vi "Write channel mapping.vi"(8 "error in (no error)":errorcluster, 11 "?":T1) -> (0 "error out":errorcluster)   [LabVIEW 2017]
uses:
  Controls/Testscreen_Input cluster.ctl
  <vilib>/addons/database/Connection.llb/Conn ObjectReference.ctl
  <vilib>/Utility/file.llb/Write Delimited Spreadsheet (string).vi
  <vilib>/addons/database/NI_Database_API.lvlib
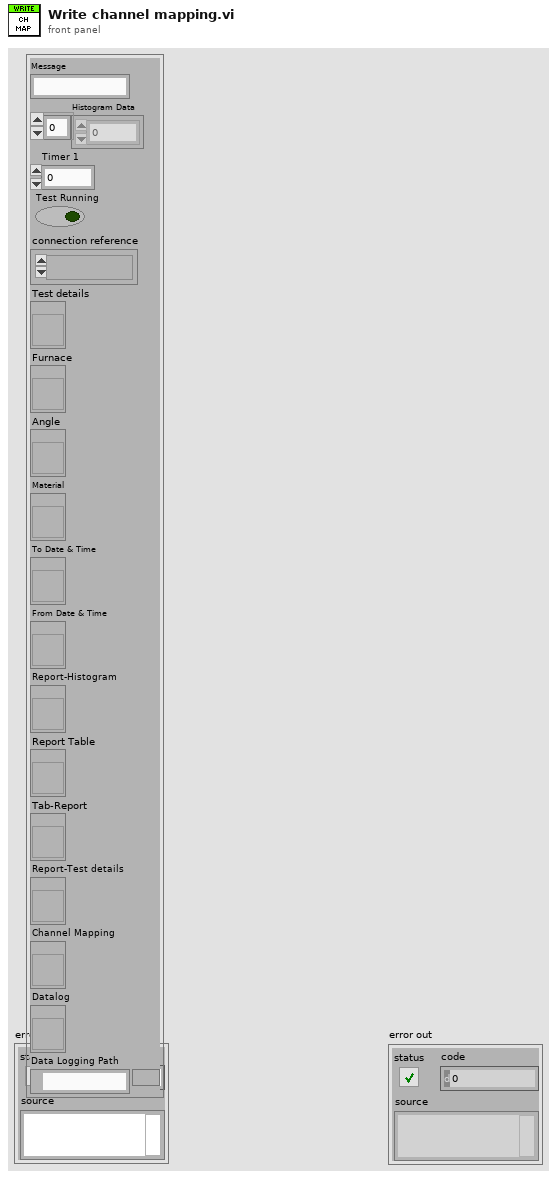
[diagram p1: front panel]
types:
  T1 = typedef "Testscreen_Input cluster.ctl" = cluster{"Message":string, "Histogram Data":i32[], "Timer 1":u32, "Test Running":bool, "connection reference":T2, "Test details":refnum<vi>, "Furnace":refnum<vi>, "Angle":refnum<vi>, "Material":refnum<vi>, "To Date & Time":refnum<vi>, "From Date & Time":refnum<vi>, "Report-Histogram":refnum<vi>, "Report Table":refnum<vi>, "Tab-Report":refnum<vi>, "Report-Test details":refnum<vi>, "Channel Mapping":refnum<vi>, "Datalog":refnum<vi>, "Data Logging Path":path}
  T2 = typedef "NI_Database_API.lvlib/Conn ObjectReference.ctl" = refnum<k1>
  T3 = cluster{"Channel Name":string, " Physical Channel":string, "Selecion?":bool}[]
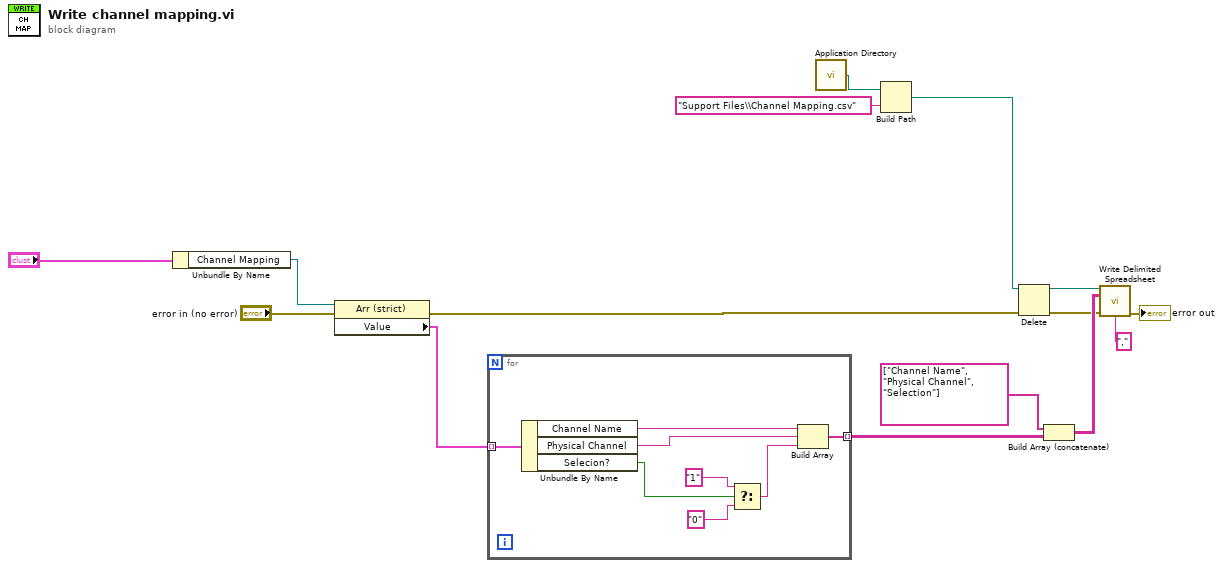
[diagram p0: block diagram]
diagram:
  n1 = Unbundle By Name("?") -> ("Channel Mapping"=w14:refnum<vi>)
  n2 = property class="Arr (strict)"(reference=w14, error in="error in (no error)") -> (error out=w2:errorcluster, "Value"=w12:T3)  [unwired: 1 out]
  n3 = for {
    tunnel: w12 -> [w23] mode=indexing
    tunnel: [w16] -> w10 mode=indexing
    n4 = Unbundle By Name(w23) -> ("Channel Name"=w19:string, "Physical Channel"=w18:string, "Selecion?"=w22:bool)
    n5 = Select(t="1", s=w22, f="0") -> (s? t:f=w17:string)
    n6 = Build Array(w19, w18, w17) -> (w16:string[])
  }
  n7 = call <vilib>:"Application Directory.vi"() -> ("Application Directory"=w9:path)
  n8 = Build Path(base path=w9, name or relative path="Support Files\\Channel Mapping.csv") -> (appended path=w4:path)
  n9 = Delete(path (use dialog)=w4, error in=w2) -> (deleted path=w3:path, error out=w1:errorcluster)  [unwired: 3 in, 1 out]
  n10 = Build Array (concatenate)(string[] ["Channel Name", "Physical Channel", "Selection"], w10) -> (w7:string[][])
  n11 = call-poly <vilib>:"Write Delimited Spreadsheet.vi"("file path (dialog if empty)"=w3, "2D data"=w7, "error in (no error)"=w1, "delimiter (\\t)"="," ("delimiter (\\t)")) -> ("error out"=→"error out":errorcluster)  [unwired: 10 in, 1 out]
